vi "DAQ_V3_ben.vi"() -> ()   [LabVIEW 2017]
panel:
  in  "TABS":enum32{"CONTROLS", "SETUP"}(tab)
  in  "End Acquisition":bool
  in  "COM Port Settings":T1={"Unit ID"="A", "Baud Rate"=enum."19200", "VISA Sesssion In"="COM1"}
  in  "Device":string="ECR Thruster"
  in  "Test Campaign":string="Junior"
  in  "User Initials":string="BNW"
  # "FILE SETUP"
  # "FLOW CONTROL"
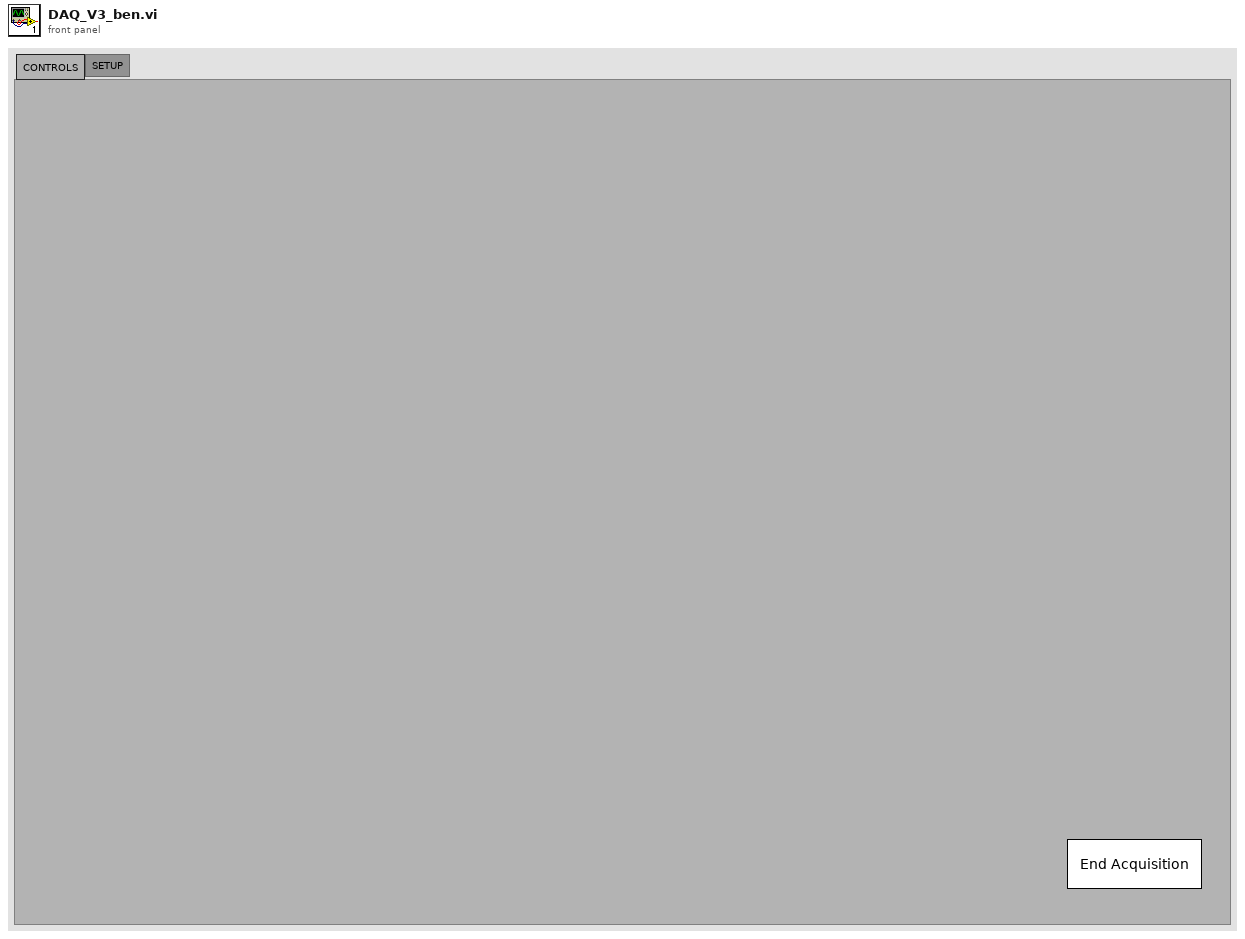
[diagram p1: front panel]
types:
  T1 = cluster{"Unit ID":string, "Baud Rate":enum8{"2400", "9600", "19200", "38400", "57600", "115200", "Unknown"}, "VISA Sesssion In":refnum<visa-resource-name>}
  T2 = cluster{"Controller Full Scale":dbl, "Controller Select":u16, "Control Range":enum16{"Normal", "Inverted", "Bidirectional", "Unknown"}}
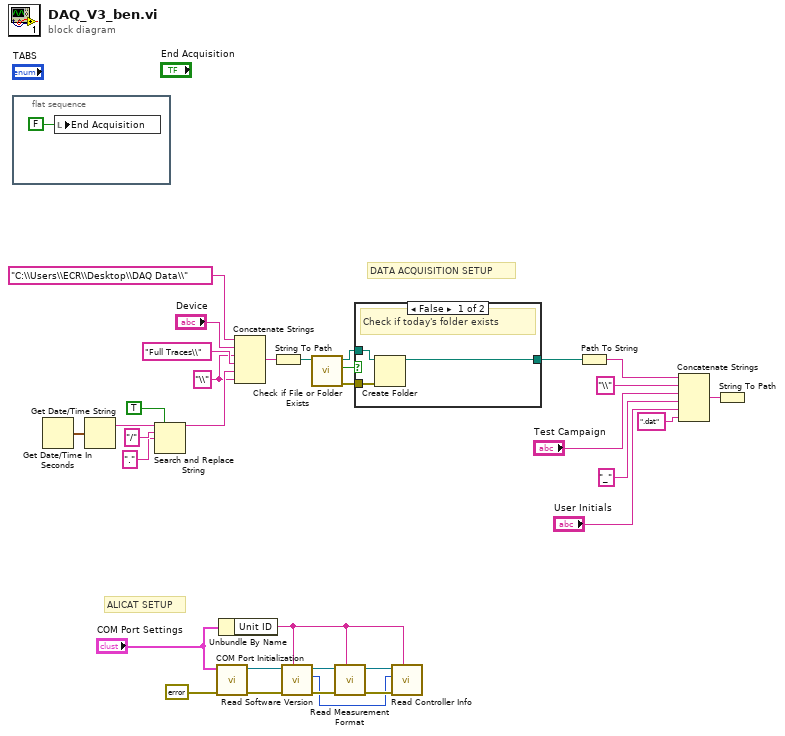
[diagram p0: block diagram]
diagram:
  w26 = "\\" ("string")
  # "ALICAT SETUP"
  # "DATA ACQUISITION SETUP"
  n1 = flat-sequence {
    frame #0 {
      n2 = local write "End Acquisition"(FALSE ("End Acquisition")) -> ()
    }
  }
  n3 = Get Date/Time In Seconds() -> (seconds since 1Jan1904=w34:timestamp)
  n4 = Get Date/Time String(seconds (now)=w34) -> (date string=w33:string)  [unwired: 2 in, 1 out]
  n5 = Search and Replace String(replace all?=TRUE ("replace all? (F)"), input string=w33, search string="/", replace string="." ("replace string (\"\")")) -> (result string=w27:string)  [unwired: 4 in, 3 out]
  n6 = call "COM Port Initialization.vi"("error in (no error)"=errorcluster {"status"=FALSE, "code"=0, "source"=""}, "Communication Settings"="COM Port Settings") -> ("error out"=w6:errorcluster, "VISA Session Out"=w7:refnum<visa-resource-name>)  [unwired: 8 in]
  n7 = Unbundle By Name("COM Port Settings") -> ("Unit ID"=w5:string)
  n8 = Concatenate Strings("C:\\Users\\ECR\\Desktop\\DAQ Data\\", "Device", w26, "Full Traces\\" ("string"), w27, w26) -> (w19:string)
  n9 = String To Path(string=w19) -> (path=w24:path)
  n10 = call "Read Software Version.vi"("Unit ID (A)"=w5, "error in"=w6, "VISA Session In"=w7) -> ("error out"=w4:errorcluster, "Software Version"=w2:u8, "VISA Session Out"=w3:refnum<visa-resource-name>)  [unwired: 6 in]
  n11 = call <vilib>:"Check if File or Folder Exists.vi"("path"=w24) -> ("error out"=w22:errorcluster, "file or folder exists?"=w21:bool, "dup path"=w23:path)  [unwired: 8 in]
  n12 = call "Read Measurement Format.vi"("Unit ID (A)"=w5, "error in"=w4, "VISA Session In"=w3) -> ("error out"=w10:errorcluster, "VISA Session Out"=w9:refnum<visa-resource-name>)  [unwired: 6 in, 1 out]
  n13 = case shown="False" w21 {
    tunnel: w23 -> [w38 w39]
    tunnel: w22 -> [w37 _]
    tunnel: [w36 w39] -> w20
    frame False {
      # "Check if today's folder exists"
      n14 = Create Folder(path (use dialog)=w38, error in=w37) -> (created path=w36:path)  [unwired: 1 in, 2 out]
    }
    frame True {
    }
  }
  n15 = call "Read Controller Info.vi"("Unit ID (A)"=w5, "error in"=w10, "Software Version"=w2, "VISA Session In"=w9) -> ("Controller Info out"=w8:T2)  [unwired: 4 in, 3 out]
  n16 = Path To String(path=w20) -> (string=w12:string)
  n17 = Concatenate Strings(w12, "\\" ("string"), "Test Campaign", "_" ("string"), "User Initials", ".dat" ("string")) -> (w18:string)
  n18 = String To Path(string=w18) -> ()  [unwired: 1 out]
